vi "0~1随机数发生器(M).vi"(8 "Error In":errorcluster caption="错误输入") -> (0 "Error Out":errorcluster caption="错误输出")   [LabVIEW 2012]
uses:
  <vilib>/imath/engines/lvmath2/RunTimeEngine/ErrorHandling/NIMS_Finalize Error.vi
  <vilib>/imath/engines/lvmath2/RunTimeEngine/NodeEndStatement/NIMS_NodeEndStatement_Get Vector.vi
  <instcachedir>/0/NIMS_NodeEndStatement_Get Vector_2BE3967F82A04EDB90B65AFAEF9E88C9.lvgen/NIMS_NodeEndStatement_Get Vector_2BE3967F82A04EDB90B65AFAEF9E88C9_001.vi
  <vilib>/imath/engines/lvmath/Functions/Error Handling/MergeErrorsWrapper.vi
  <vilib>/imath/engines/lvmath2/RunTimeEngine/NodeEndStatement/NIMS_NodeEndStatement_Output.vi
  <instcachedir>/0/NIMS_NodeEndStatement_Output_53EC0D466D134D7ABD903AC30B43404B.lvgen/NIMS_NodeEndStatement_Output_53EC0D466D134D7ABD903AC30B43404B_002.vi
  <instcachedir>/0/NIMS_NodeEndStatement_Output_53EC0D466D134D7ABD903AC30B43404B.lvgen/NIMS_NodeEndStatement_Output_53EC0D466D134D7ABD903AC30B43404B_005.vi
  <instcachedir>/0/NIMS_NodeEndStatement_Output_53EC0D466D134D7ABD903AC30B43404B.lvgen/NIMS_NodeEndStatement_Output_53EC0D466D134D7ABD903AC30B43404B_001.vi
  <vilib>/imath/engines/lvmath2/RunTimeEngine/BuiltInFunctions/rand/NIMS_rand().vi
  <vilib>/imath/engines/lvmath2/RunTimeEngine/ErrorHandling/NIMS_Error From Error Code.vi
  <vilib>/imath/engines/lvmath2/RunTimeEngine/BuiltInFunctions/rand/NIMS_rand(I32).vi
  <vilib>/imath/engines/lvmath2/RunTimeEngine/BuiltInFunctions/rand/NIMS_rand(I32,I32).vi
panel:
  out "Rand_1D_dbl":dbl[](array[numeric])
  out "Rand_2D_dbl":dbl[][](array[numeric])
  out "Rand_dbl":dbl
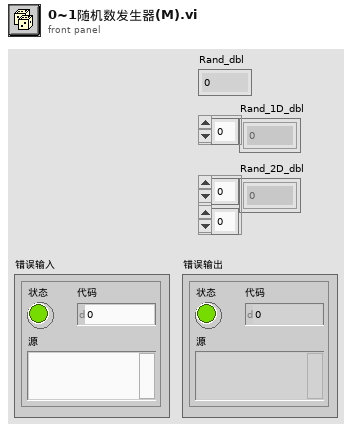
[diagram p1: front panel]
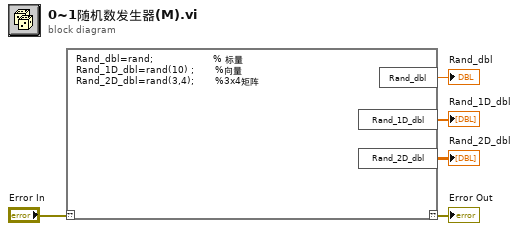
[diagram p0: block diagram]
diagram:
  n1 = mathscript code="Rand_dbl=rand;                    % 标量\nRand_1D_dbl=rand(10) ;       %向量\nRand_2D_dbl=rand(3,4);       %3x4矩阵"("??"="Error In") -> ("??"=→"Error Out":errorcluster, "Rand_dbl"=→"Rand_dbl":dbl, "Rand_1D_dbl"=→"Rand_1D_dbl":dbl[], "Rand_2D_dbl"=→"Rand_2D_dbl":dbl[][])
